vi "To robot frame.vi"(10 "Odometry":T1, 11 "Lookahead Point":T2) -> (3 "Lookahead Point Out":cluster{"x out":dbl, "y out":dbl})   [LabVIEW 2017, in "Pure Pursuit.lvlib"]
uses:
  Pure Pursuit.lvlib
  Typedef/Path Point.ctl
  Odometry/Typedef/Odometry.ctl
  <vilib>/Analysis/coordinate.llb/2D Cartesian Coordinate Shift (Scalar).vi
  <vilib>/Analysis/coordinate.llb/2D Cartesian Coordinate Rotation (Scalar).vi
  <vilib>/Analysis/NI_AALPro.lvlib
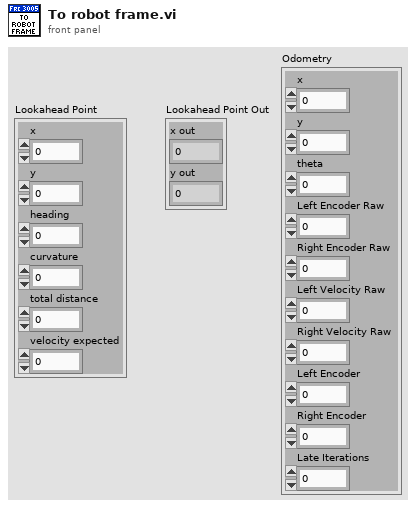
[diagram p1: front panel]
types:
  T1 = typedef "Odometry.ctl" = cluster{"x":dbl, "y":dbl, "theta":dbl, "Left Encoder Raw":i32, "Right Encoder Raw":i32, "Left Velocity Raw":i32, "Right Velocity Raw":i32, "Left Encoder":dbl, "Right Encoder":dbl, "Late Iterations":i16}
  T2 = typedef "Pure Pursuit.lvlib/Path Point.ctl" = cluster{"x":dbl, "y":dbl, "heading":dbl, "curvature":dbl, "total distance":dbl, "velocity expected":dbl}
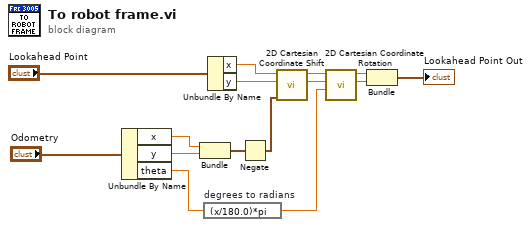
[diagram p0: block diagram]
diagram:
  n1 = Unbundle By Name("Odometry") -> ("x"=w13:dbl, "y"=w12:dbl, "theta"=w14:dbl)
  n2 = Bundle("x"=w13, "y"=w12) -> (w7:cluster{"x":dbl, "y":dbl})  [unwired: 1 in]
  n3 = expression code="(x/180.0)*pi" "degrees to radians"(w14) -> (w15:dbl)
  n4 = Unbundle By Name("Lookahead Point") -> ("x"=w5:dbl, "y"=w6:dbl)
  n5 = Negate(x=w7) -> (-x=w8:cluster{"x":dbl, "y":dbl})
  n6 = call-poly <vilib>:"2D Cartesian Coordinate Shift.vi"("shift"=w8, "y"=w6, "x"=w5) -> ("y out"=w3:dbl, "x out"=w2:dbl)  [unwired: 6 in, 1 out]
  n7 = call-poly <vilib>:"2D Cartesian Coordinate Rotation.vi"("theta"=w15, "y"=w3, "x"=w2) -> ("y out"=w9:dbl, "x out"=w10:dbl)  [unwired: 6 in, 1 out]
  n8 = Bundle("x out"=w10, "y out"=w9) -> (→"Lookahead Point Out":cluster{"x out":dbl, "y out":dbl})  [unwired: 1 in]
